vi "myXi_GetParameter.vi"(7 "input PRM":T3, 8 "error in":errorcluster, 11 "xiCam IN":refnum<k24>) -> (0 "error out":errorcluster, 1 "Type":T2, 2 "Method":T1, 3 "xiCam Out":refnum<k24>, 4 "output":variant, 6 "Desc.":string)   [LabVIEW 2018]
uses:
  VisionLibrariesXimea/xiLib/xiLIB_64bit/xiLIB/xiCamLib/xiCam/PRM/PRM/PRM_v2.ctl
  C:/XIMEA/API/x64/xiApi.NETX64.dll
  VisionLibrariesXimea/xiLib/xiLIB_64bit/xiLIB/xiCamLib/xiLIB/Typedefs/xiLIB - PRM_Type.ctl
  VisionLibrariesXimea/xiLib/xiLIB_64bit/xiLIB/xiCamLib/xiLIB/Typedefs/xiLIB - PRM_Function.ctl
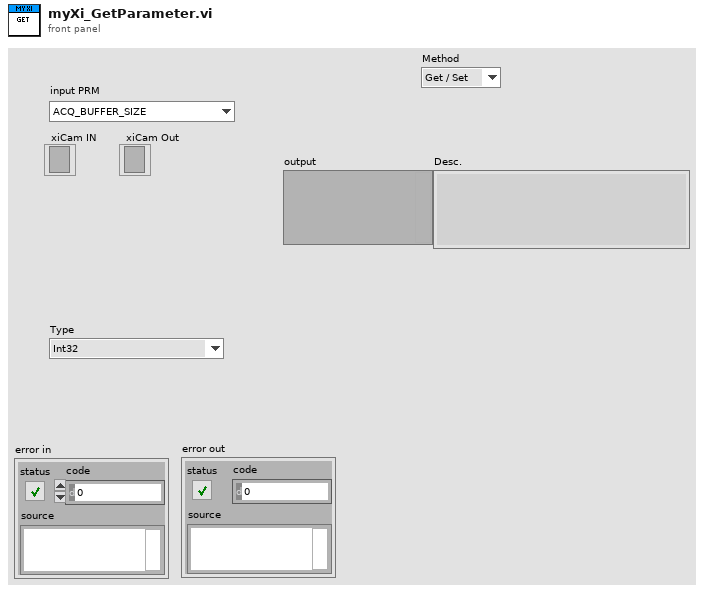
[diagram p1: front panel]
types:
  T1 = typedef "xiLIB - PRM_Function.ctl" = enum16{"Get / Set", "Get", "Set"}
  T2 = typedef "xiLIB - PRM_Type.ctl" = enum16{"Int32", "Float", "String", "DOWNSAMPLING_TYPE", "IMAGE_DATA_FORMAT", "BUFFER_POLICY", "TRG_SOURCE", "GPI", "GPO", "ACQ_TIMING_MODE", "BINNING_PATTERN", "BINNING_SELECTOR", "CMS_MODE", "COUNTER_SELECTOR", "DEBUG_LEVEL", "DECIMATION_PATTERN", "DECIMATION_SELECTOR", "GAIN_SELECTOR_TYPE", "LED_MODE", "LENS_FEATURE_SELECTOR", "LENS_MODE", "OUTPUT_DATA_PACKING_TYPE", "SENSOR_FEATURE_SELECTOR", "SHUTTER_TYPE", "TRG_SELECTOR", "TS_RST_MODE", "TS_RST_SOURCE"}
  T3 = typedef "PRM_v2.ctl" = enum16{"ACQ_BUFFER_SIZE", "ACQ_FRAME_BURST_COUNT", "ACQ_TIMING_MODE", "ACQ_TRANSPORT_BUFFER_SIZE", "AE_MAX_LIMIT", "AEAG", "AEAG_LEVEL", "API_VERSION", "AG_MAX_LIMIT", "APPLY_CMS", "AUTO_BANDWIDTH_CALCULATION", "AUTO_WB", "AVAILABLE_BANDWIDTH", "AVAILABLE_BANDWIDTH_MAX", "AVAILABLE_BANDWIDTH_MIN", "BPC", "BUFFER_POLICY", "BUFFERS_QUEUE_SIZE", "CC_MATRIX_00", "CC_MATRIX_01", "CC_MATRIX_02", "CC_MATRIX_03", "CC_MATRIX_10", "CC_MATRIX_11", "CC_MATRIX_12", "CC_MATRIX_13", "CC_MATRIX_20", "CC_MATRIX_21", "CC_MATRIX_22", "CC_MATRIX_23", "CC_MATRIX_30", "CC_MATRIX_31", "CC_MATRIX_32", "CC_MATRIX_33", "CHIP_TEMP", "CMS", "COLOR_FILTER_ARRAY", "COOLING", "DEBOUNCE_EN", "DEBOUNCE_POL", "DEBOUNCE_T0", "DEBOUNCE_T1", "DEBUG_LEVEL", "DEFAULT_CC_MATRIX", "DEVICE_INSTANCE_PATH", "DEVICE_MODEL_ID", "DEVICE_NAME", "DEVICE_SN", "DEVICE_TYPE", "DEVICE_USER_ID", "DOWNSAMPLING", "DOWNSAMPLING_MAX", "DOWNSAMPLING_MIN", "DOWNSAMPLING_TYPE", "DRV_VERSION", "EXP_PRIORITY", "EXPOSURE", "EXPOSURE_DIRECT_UPDATE", "EXPOSURE_MAX", "EXPOSURE_MIN", "FFS_FILE_NAME", "FPGA1_VERSION", "FRAMERATE", "FRAMERATE_MAX", "FRAMERATE_MIN", "FREE_FFS_SIZE", "GAIN", "GAIN_DIRECT_UPDATE", "GAIN_MAX", "GAIN_MIN", "GAMMAC", "GAMMAY", "GPI_LEVEL", "GPI_MODE", "GPI_SELECTOR", "GPI_SELECTOR_MAX", "GPI_SELECTOR_MIN", "GPO_MODE", "GPO_SELECTOR", "GPO_SELECTOR_MAX", "GPO_SELECTOR_MIN", "HDR", "HDR_T1", "HDR_T2", "HEIGHT", "HEIGHT_MAX", "HEIGHT_MIN", "HOUSE_TEMP", "IMAGE_DATA_FORMAT", "IMAGE_IS_COLOR", "INPUT_CMS_PROFILE", "IS_COOLED", "IS_DEVICE_EXIST", "KNEEPOINT1", "KNEEPOINT2", "LED_MODE", "LED_SELECTOR", "LED_SELECTOR_MAX", "LED_SELECTOR_MIN", "LIMIT_BANDWIDTH", "LIMIT_BANDWIDTH_MAX", "LIMIT_BANDWIDTH_MIN", "LUT_EN", "LUT_INDEX", "LUT_INDEX_MAX", "LUT_INDEX_MIN", "LUT_VALUE", "LUT_VALUE_MAX", "LUT_VALUE_MIN", "MANUAL_WB", "MCU1_VERSION", "MCU2_VERSION", "OFFSET_X", "OFFSET_X_MAX", "OFFSET_X_MIN", "OFFSET_Y", "OFFSET_Y_MAX", "OFFSET_Y_MIN", "OUTPUT_CMS_PROFILE", "OUTPUT_DATA_BIT_DEPTH", "OUTPUT_DATA_PACKING", "READ_FILE_FFS", "RECENT_FRAME", "SENSOR_DATA_BIT_DEPTH", "SENSOR_MODE", "SENSOR_TAPS", "SHARPNESS", "SHUTTER_TYPE", "TARGET_TEMP", "TRG_DELAY", "TRG_SELECTOR", "TRG_SOFTWARE", "TRG_SOURCE", "USED_FFS_SIZE", "WB_KB", "WB_KG", "WB_KR", "WIDTH", "WIDTH_MAX", "WIDTH_MIN", "WRITE_FILE_FFS", "ACQ_BUFFER_SIZE_UNIT", "ACQ_TRANSPORT_BUFFER_COMMIT", "AEAG_ROI_HEIGHT", "AEAG_ROI_OFFSET_X", "AEAG_ROU_OFFSET_Y", "AEAG_ROI_WIDTH", "API_CONTEXT_LIST", "BINNING_HORIZONTAL", "BINNING_SELECTOR", "BINNING_VERTICAL", "COLUMN_FPN_CORRECTION", "COUNTER_SELECTOR", "COUNTER_VALUE", "DECIMATION_HORIZONTAL", "DECIMATION_SELECTOR", "DECIMATION_VERTICAL", "DEVICE_ID", "DEVICE_LOCATION_PATH", "DEVICE_MANIFEST", "DEVICE_RESET", "DEVICE_SENS_SN", "EXPOSURE_BURST_COUNT", "FFS_ACCESS_KEY", "GAIN_SELECTOR", "HW_REVISION", "IMAGE_BLACK_LEVEL", "IMAGE_DATA_BIT_DEPTH", "IMAGE_DATA_FORMAT_RGB32_ALPHA", "IMAGE_PAYLOAD_SIZE", "LENS_APERTURE_VALUE", "LENS_FEATURE", "LENS_FEATURE_SELECTOR", "LENS_FOCAL_LENGTH", "LENS_FOCUS_DISTANCE", "LENS_FOCUS_MOVE", "LENS_FOCUS_MOVEMENT_VALUE", "LENS_MODE", "OUTPUT_DATA_PACKING_TYPE", "SENSOR_CLOCK_FREQ_HZ", "SENSOR_CLOCK_FREQ_INDEX", "SENSOR_FEATURE_SELECTOR", "SENSOR_FEATURE_VALUE", "SENSOR_OUTPUT_CHANNEL_COUNT", "TRANSPORT_PIXEL_FORMAT", "TS_RST_MODE", "TS_RST_SOURCE"}
  T4 = typedef "xiLIB - PRM_Attribute.ctl" = cluster{"Type":T2, "Method":T1, "Desc.":string, "PRM":T3}
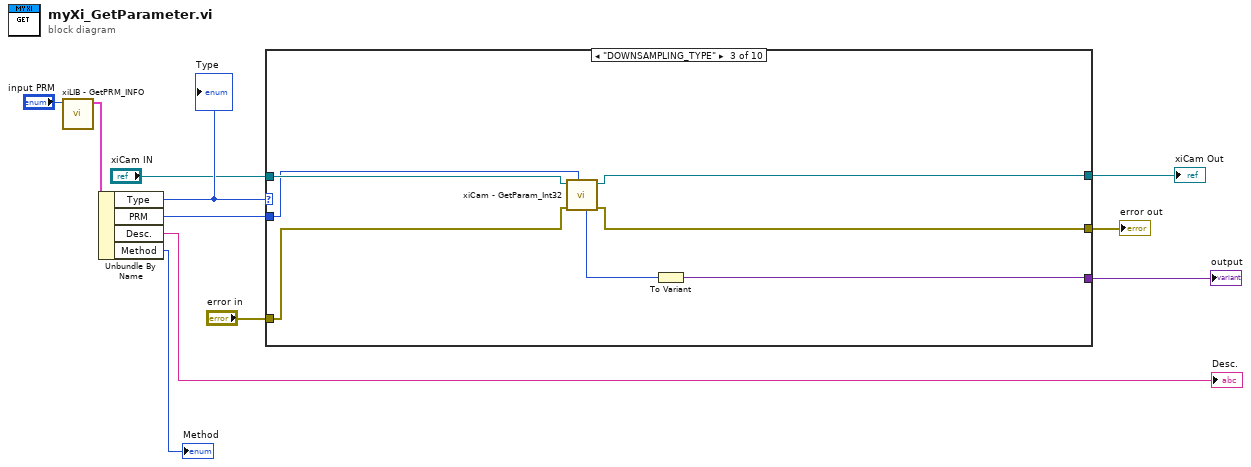
[diagram p0: block diagram]
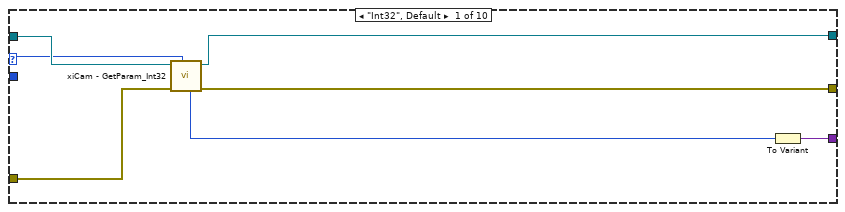
[diagram p2: hidden frame]
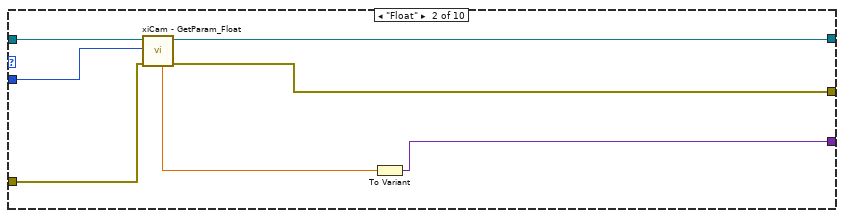
[diagram p3: hidden frame]
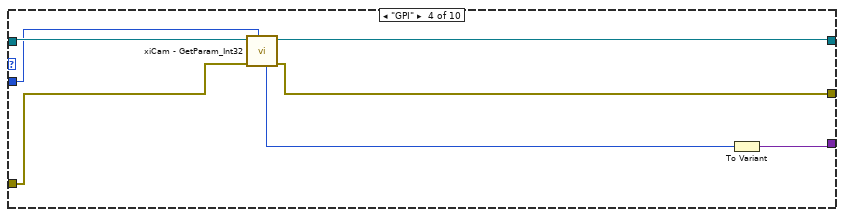
[diagram p4: hidden frame]
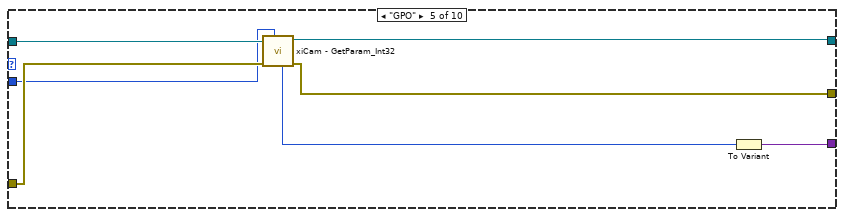
[diagram p5: hidden frame]
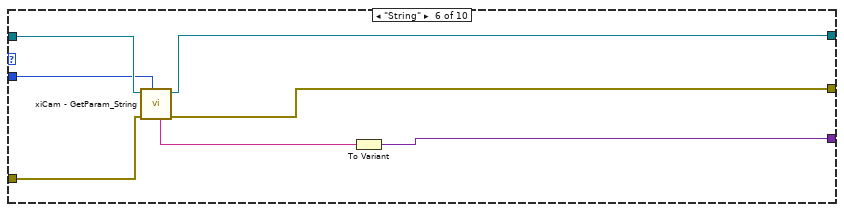
[diagram p6: hidden frame]
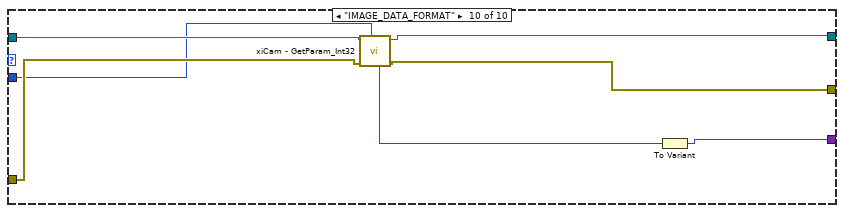
[diagram p10: hidden frame]
diagram:
  n1 = call "xiLIB - GetPRM_INFO.vi"("PRM"="input PRM") -> ("PRM_Attributes"=w10:T4)  [unwired: 10 in]
  n2 = Unbundle By Name(w10) -> ("Type"=w9:T2, "PRM"=w7:T3, "Desc."=→"Desc.":string, "Method"=→"Method":T1)
  "Type" <- w9
  n3 = case shown="\"DOWNSAMPLING_TYPE\"" w9 {
    tunnel: "xiCam IN" -> [w15 w25 w32 w39 w46 w53 w55 w57 w59 w62]
    tunnel: w7 -> [w14 w24 w27 w37 w42 w52 _ _ _ w60]
    tunnel: [w12 w23 w29 w38 w45 w51 w55 w57 w59 w61] -> w6
    tunnel: [w13 w22 w30 w35 w43 w47 w54 w56 w58 w63] -> w5
    tunnel: [w17 w20 w28 w34 w41 w49 _ _ _ w66] -> w3
    tunnel: "error in" -> [w16 w19 w31 w36 w44 w48 w54 w56 w58 w64]
    frame "Int32", Default {
      n4 = call "xiCam - GetParam_Int32.vi"("PRM"=w14, "error in (no error)"=w16, "xiCam In"=w15) -> ("error out"=w13:errorcluster, "xiCam Out"=w12:refnum<k24>, "Int32_Value"=w18:i32)  [unwired: 6 in]
      n5 = To Variant(anything=w18) -> (Variant=w17:variant)
    }
    frame "Float" {
      n6 = call "xiCam - GetParam_Float.vi"("PRM"=w24, "error in (no error)"=w19, "xiCam In"=w25) -> ("error out"=w22:errorcluster, "xiCam Out"=w23:refnum<k24>, "Float_Value"=w21:sgl)  [unwired: 6 in]
      n7 = To Variant(anything=w21) -> (Variant=w20:variant)
    }
    frame "DOWNSAMPLING_TYPE" {
      n8 = call "xiCam - GetParam_Int32.vi"("PRM"=w27, "error in (no error)"=w31, "xiCam In"=w32) -> ("error out"=w30:errorcluster, "xiCam Out"=w29:refnum<k24>, "Int32_Value"=w26:i32)  [unwired: 6 in]
      n9 = To Variant(anything=w26) -> (Variant=w28:variant)
    }
    frame "GPI" {
      n10 = call "xiCam - GetParam_Int32.vi"("PRM"=w37, "error in (no error)"=w36, "xiCam In"=w39) -> ("error out"=w35:errorcluster, "xiCam Out"=w38:refnum<k24>, "Int32_Value"=w33:i32)  [unwired: 6 in]
      n11 = To Variant(anything=w33) -> (Variant=w34:variant)
    }
    frame "GPO" {
      n12 = call "xiCam - GetParam_Int32.vi"("PRM"=w42, "error in (no error)"=w44, "xiCam In"=w46) -> ("error out"=w43:errorcluster, "xiCam Out"=w45:refnum<k24>, "Int32_Value"=w40:i32)  [unwired: 6 in]
      n13 = To Variant(anything=w40) -> (Variant=w41:variant)
    }
    frame "String" {
      n14 = call "xiCam - GetParam_String.vi"("PRM"=w52, "error in (no error)"=w48, "xiCam In"=w53) -> ("error out"=w47:errorcluster, "xiCam Out"=w51:refnum<k24>, "String_Value"=w50:string)  [unwired: 6 in]
      n15 = To Variant(anything=w50) -> (Variant=w49:variant)
    }
    frame "ACQ_TIMING_MODE" {
    }
    frame "BINNING_PATTERN" {
    }
    frame "BINNING_SELECTOR" {
    }
    frame "IMAGE_DATA_FORMAT" {
      n16 = call "xiCam - GetParam_Int32.vi"("PRM"=w60, "error in (no error)"=w64, "xiCam In"=w62) -> ("error out"=w63:errorcluster, "xiCam Out"=w61:refnum<k24>, "Int32_Value"=w65:i32)  [unwired: 6 in]
      n17 = To Variant(anything=w65) -> (Variant=w66:variant)
    }
  }
  "xiCam Out" <- w6
  "output" <- w3
  "error out" <- w5
